vi "testPictureOverNetwork.vi"() -> ()   [LabVIEW 2009, in "run.lvlib"]
uses:
  testing/run.lvlib
panel:
  in  "address":string="192.168.104.186"
  in  "Machine":enum16{"Local", "Network"}(ring)=enum."Network"
  out "pictures recieved":i32
  out "error out":errorcluster
  in  "stop":bool
  out "value":T1(plugin-control)
  # "client start after server"
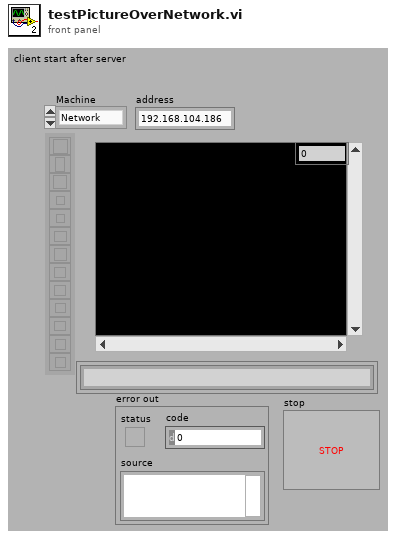
[diagram p1: front panel]
types:
  T1 = typedef "IMAQ Image.ctl" = refnum<image>
  T2 = cluster{"Message":enum16{"Idle", "initialise", "configureAcquisition", "setTemperature", "getTemperature", "start", "stop", "sendImage", "close", "error", "ExitApp"}, "Data":variant}
  T3 = enum16{"Idle", "initialise", "configureAcquisition", "setTemperature", "getTemperature", "start", "stop", "sendImage", "close", "error", "ExitApp"}
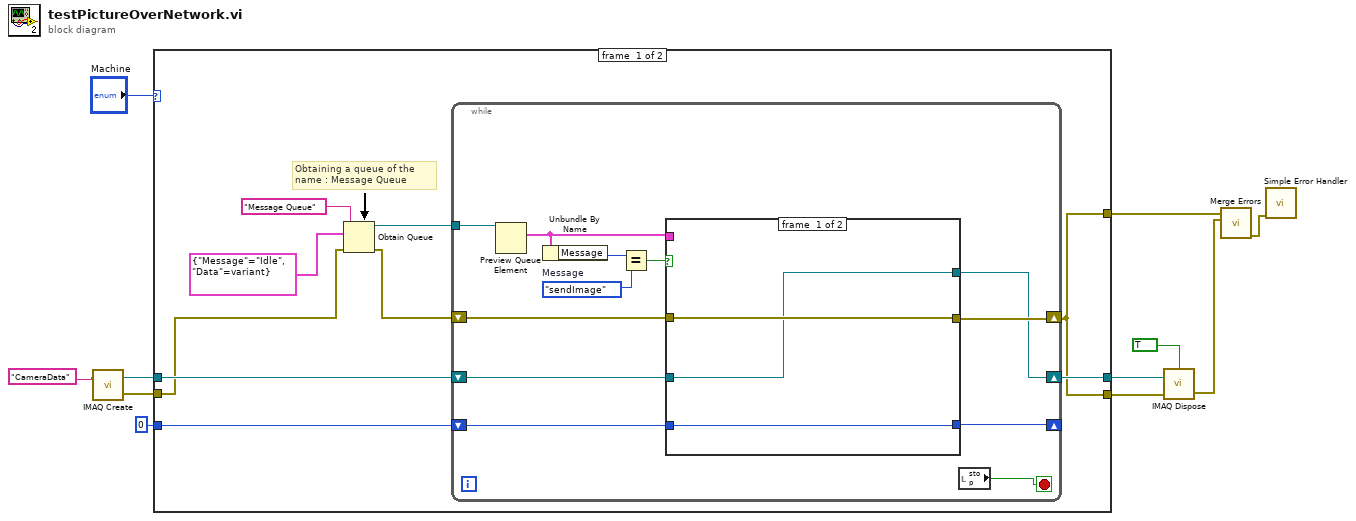
[diagram p0: block diagram]
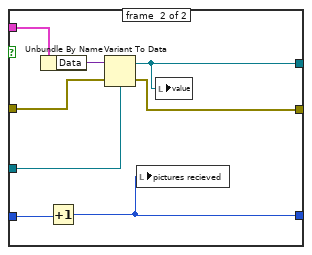
[diagram p2: hidden frame]
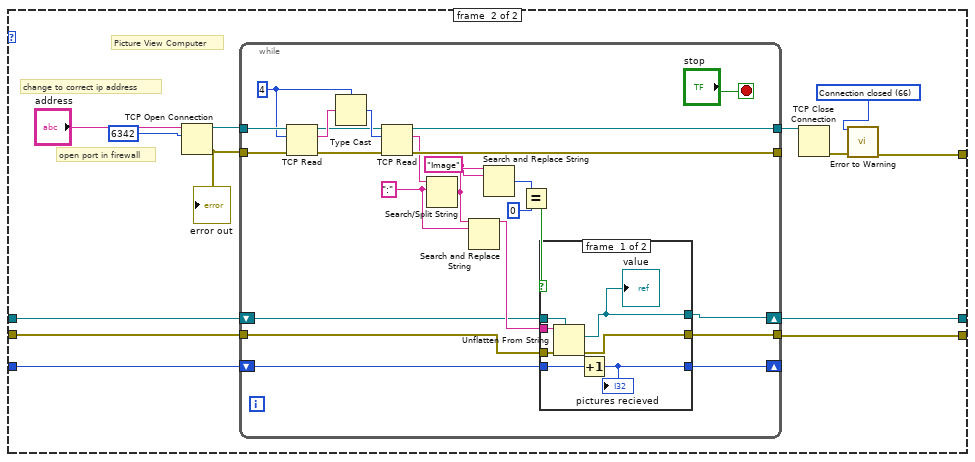
[diagram p3: hidden frame]
diagram:
  n1 = call "IMAQ Create"("Image Name"="CameraData" ("Port")) -> ("New Image"=w11:T1, "error out"=w10:errorcluster)  [unwired: 4 in]
  n2 = case shown="\"Network\"" "Machine" {
    tunnel: [w14 w53] -> w3
    tunnel: w11 -> [w17 w50]
    tunnel: w10 -> [w13 w49]
    tunnel: [w16 w48] -> w8
    tunnel: [w14 w47] -> w7
    tunnel: 0 -> [w15 w45]
    frame #0 {
      # "Obtaining a queue of the name : Message Queue"
      n3 = Obtain Queue(name (unnamed)="Message Queue" ("Queue Name"), element data type=T2 {"Message"=enum."Idle", "Data"=variant}, error in (no error)=w13) -> (queue out=w18:refnum<queue>, error out=w12:errorcluster)  [unwired: 2 in, 1 out]
      n4 = while {
        tunnel: w18 -> [w32]
        shift-right: [w24] -> w16
        shift-left: w17 -> [w27]
        shift-right: [w25] -> w14
        shift-left: w12 -> [w26]
        shift-right: [w22] -> _
        shift-left: w15 -> [w23]
        stop <- w21 stop-if-true
        w30 = T3."sendImage"  # Message
        n5 = Preview Queue Element(queue=w32) -> (element=w28:T2)  [unwired: 2 in, 3 out]
        n6 = Unbundle By Name(w28) -> ("Message"=w31:T3)
        n7 = Equal?(x=w31, y=w30) -> (x = y?=w29:bool)
        n8 = case shown="True" w29 {
          tunnel: w28 -> [_ w43]
          tunnel: w27 -> [w34 w41]
          tunnel: w26 -> [w35 w40]
          tunnel: [w35 w39] -> w25
          tunnel: [w34 w38] -> w24
          tunnel: w23 -> [w33 w37]
          tunnel: [w33 w36] -> w22
          frame #0 {
          }
          frame #1 {
            n9 = Unbundle By Name(w43) -> ("Data"=w42:variant)
            n10 = Increment(x=w37) -> (x+1=w36:i32)
            n11 = Variant To Data(error in=w40, Variant=w42, type=w41) -> (error out=w39:errorcluster, data=w38:T1)
            n12 = local write "pictures recieved"(w36) -> ()
            n13 = local write "value"(w38) -> ()
          }
        }
        n14 = local read "stop"() -> (w21:bool)
      }
    }
    frame #1 {
      w52 = 66 items=["No Error", "Argument Error", "Memory Full", "Out of Zone", "End of File", "File Already Open", "Generic File IO Error", "File Not Found", "File Permission Error", "Disk Full", "Duplicate Path", "Too Many Files Open", "Not Enabled", "Resource File Not Found", "Cannot Add Resource", "Resource Not Found", "Image Not Found", "Image Memory Error", "Pen Does Not Exist", "Config Bad Type", "Config Token Not Found", "Config Parse Error", "Config Memory Error", "Bad External Code Format", "Bad External Code Offset", "External Code Not Present", "Null Window", "Destroy Window Mixup", "Null Menu", "Print Aborted", "Bad Print Record", "Print Driver Error", "Windows Error During Print", "Memory Error During Print", "Print Dialog Error", "Generic Print Error", "Invalid Device Refnum", "Device Not Found", "Device Parameter Error", "Device Unit Error", "Can't Open Device", "Device Call Aborted", "Generic Error", "Cancelled By User", "Object ID Too Low", "Object ID Too High", "Object Not In Heap", "Unknown Heap", "Bad DefProc ID", "DefProc Not In Table", "Message Out Of Range", "Null Method", "Unknown Message", "Manager Call Not Supported", "Bad address", "Connection In progress", "Connection timed out", "Connection is already in progress", "Network attribute not supported", "Network error", "Address in use", "System out of memory", "Connection aborted", "Connection refused", "Connection is not connected", "Connection is already connected", "Connection closed", "Initialize error (interapplication manager)", "Bad occurrence", "Wait on unbound occurrence handler", "Occurrence queue overflow", "Bad path", "Semaphore not signaled", "Unrecognized type (interapplication manager)"] ("1st Error to Convert")
      # "open port in firewall"
      # "change to correct ip address"
      # "Picture View Computer"
      n15 = TCP Open Connection(address="address", remote port or service name=u16 6342) -> (connection ID=w56:refnum<k5>, error out=w55:errorcluster)  [unwired: 1 in, 2 out]
      "error out" <- w55
      n16 = while {
        tunnel: [w73] -> w51
        tunnel: [w72] -> _
        tunnel: w55 -> [w79]
        tunnel: w56 -> [w80]
        tunnel: w49 -> [w70]
        tunnel: [w69] -> w47
        shift-right: [w66] -> _
        shift-left: w45 -> [w65]
        shift-right: [w63] -> w48
        shift-left: w50 -> [w64]
        stop <- "stop" stop-if-true
        w71 = ":"
        w78 = 4
        n17 = TCP Read(connection ID=w80, bytes to read=w78, error in (no error)=w79) -> (connection ID out=w74:refnum<k5>, data out=w77:string, error out=w76:errorcluster)  [unwired: 1 in, 1 out]
        n18 = Type Cast(type=w78, x=w77) -> (*(type *) &x=w75:i32)
        n19 = TCP Read(connection ID=w74, bytes to read=w75, error in (no error)=w76) -> (connection ID out=w73:refnum<k5>, data out=w62:string, error out=w72:errorcluster)  [unwired: 1 in, 1 out]
        n20 = Search/Split String(string=w62, search string/char (-)=w71) -> (match + rest of string=w61:string)  [unwired: 1 in, 2 out]
        n21 = Search and Replace String(input string=w61, search string=w71) -> (result string=w67:string)  [unwired: 6 in, 3 out]
        n22 = Search and Replace String(input string=w61, search string="Image") -> (number of replacements=w59:i32)  [unwired: 6 in, 3 out]
        n23 = Equal?(x=w59, y=0) -> (x = y?=w57:bool)
        n24 = case shown="False" w57 {
          tunnel: w70 -> [w87 w90]
          tunnel: [w86 w90] -> w69
          tunnel: w64 -> [w85 w88]
          tunnel: w67 -> [w84 _]
          tunnel: [w83 w89] -> w66
          tunnel: w65 -> [w82 w89]
          tunnel: [w81 w88] -> w63
          frame #0 {
            n25 = Unflatten From String(type=w85, binary string=w84, error in (no error)=w87) -> (value=w81:T1, error out=w86:errorcluster)  [unwired: 2 in, 1 out]
            "value" <- w81
            n26 = Increment(x=w82) -> (x+1=w83:i32)
            "pictures recieved" <- w83
          }
          frame #1 {
          }
        }
      }
      n27 = TCP Close Connection(connection ID=w51) -> (error out=w54:errorcluster)  [unwired: 1 in, 2 out]
      n28 = call <vilib>:"Error to Warning.vi"("1st Error to Convert"=w52, "error in"=w54) -> ("warning out"=w53:errorcluster)  [unwired: 3 in, 10 out]
    }
  }
  n29 = call "IMAQ Dispose"("All Images? (No)"=TRUE, "Image"=w8, "error in (no error)"=w7) -> ("error out"=w2:errorcluster)  [unwired: 3 in]
  n30 = call <vilib>:"Merge Errors.vi"("error in 2 (no error)"=w2, "error in 1 (no error)"=w3) -> ("error out"=w4:errorcluster)  [unwired: 5 in]
  n31 = call <vilib>:"Simple Error Handler.vi"("error in (no error)"=w4) -> ()  [unwired: 1 in, 8 out]
